vi "valve_test.vi"() -> ()   [LabVIEW 2020]
uses:
  istr.lib/Agilent 33XXX Series/Agilent 33XXX Series.lvlib
panel:
  out "error out":errorcluster
  in  "Amplitude (1)":dbl=1.0
  in  "VISA resource name":refnum<visa-resource-name>
  out "Status":bool
  in  "Interval (s)":dbl
  out "Cycle #":i32
  in  "stop":bool
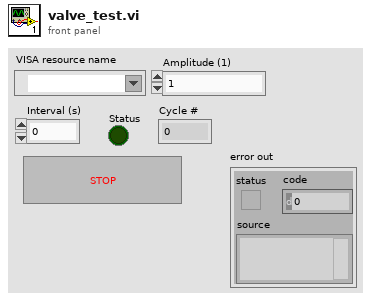
[diagram p1: front panel]
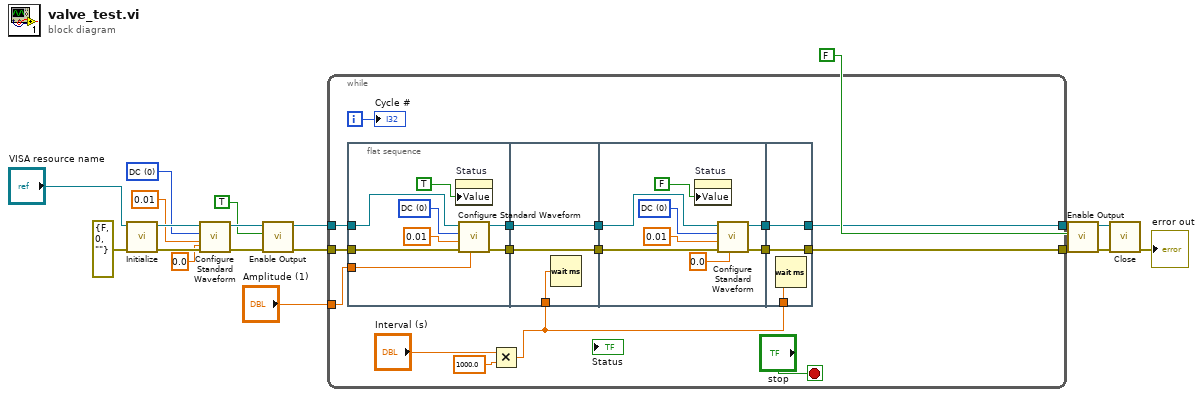
[diagram p0: block diagram]
diagram:
  w13 = u16 0 items=["DC", "Sine", "Square", "Triangle", "Ramp", "Pulse", "Noise", "Sinc", "Negative Ramp", "Exponential Rise", "Exponential Fall", "Cardiac"] ("Waveform Function (1: Sine)")
  n1 = call "Initialize.vi"("error in (no error)"=errorcluster {"status"=FALSE, "code"=0, "source"=""}, "VISA resource name"="VISA resource name") -> ("error out"=w17:errorcluster, "VISA resource name out"=w18:refnum<visa-resource-name>)  [unwired: 8 in]
  n2 = call "Configure Standard Waveform.vi"("DC Offset (0.00 V)"=0.0, "error in (no error)"=w17, "Amplitude (1)"=0.01, "Waveform Function (1: Sine)"=w13, "VISA resource name"=w18) -> ("error out"=w9:errorcluster, "VISA resource name out"=w10:refnum<visa-resource-name>)  [unwired: 5 in]
  n3 = call "Enable Output.vi"("error in (no error)"=w9, "Enable Output  (T: Enable)"=TRUE, "VISA resource name"=w10) -> ("error out"=w6:errorcluster, "VISA resource name out"=w7:refnum<visa-resource-name>)  [unwired: 7 in]
  n4 = while {
    tunnel: "Amplitude (1)" -> [w29]
    tunnel: w7 -> [w28]
    tunnel: w6 -> [w27]
    tunnel: [w24] -> w5
    tunnel: [w23] -> w4
    i -> [w35]
    stop <- "stop" stop-if-true
    n5 = flat-sequence {
      tunnel: [w42] -> w31
      tunnel: w29 -> [w41]
      tunnel: w28 -> [w40]
      tunnel: w27 -> [w39]
      tunnel: [w38] -> w25
      tunnel: w20 -> [w46]
      tunnel: w31 -> [w45]
      tunnel: [w45] -> w30
      tunnel: [w44] -> w26
      tunnel: w25 -> [w44]
      tunnel: w30 -> [w53]
      tunnel: w26 -> [w52]
      tunnel: [w50] -> w22
      tunnel: [w49] -> w21
      tunnel: [w56] -> w23
      tunnel: [w57] -> w24
      tunnel: w22 -> [w57]
      tunnel: w21 -> [w56]
      tunnel: w20 -> [w55]
      frame #0 {
        w36 = u16 0 items=["DC", "Sine", "Square", "Triangle", "Ramp", "Pulse", "Noise", "Sinc", "Negative Ramp", "Exponential Rise", "Exponential Fall", "Cardiac"] ("Waveform Function (1: Sine)")
        n6 = property on="Status" class="Bool (strict)"("Value"=TRUE ("Enable Output  (T: Enable)")) -> ()  [unwired: 2 in, 2 out]
        n7 = call "Configure Standard Waveform.vi"("DC Offset (0.00 V)"=w41, "error in (no error)"=w39, "Amplitude (1)"=0.01, "Waveform Function (1: Sine)"=w36, "VISA resource name"=w40) -> ("error out"=w42:errorcluster, "VISA resource name out"=w38:refnum<visa-resource-name>)  [unwired: 5 in]
      }
      frame #1 {
        n8 = Wait (ms)(milliseconds to wait=w46) -> ()  [unwired: 1 out]
      }
      frame #2 {
        w48 = u16 0 items=["DC", "Sine", "Square", "Triangle", "Ramp", "Pulse", "Noise", "Sinc", "Negative Ramp", "Exponential Rise", "Exponential Fall", "Cardiac"] ("Waveform Function (1: Sine)")
        n9 = property on="Status" class="Bool (strict)"("Value"=FALSE ("Enable Output  (T: Enable)")) -> ()  [unwired: 2 in, 2 out]
        n10 = call "Configure Standard Waveform.vi"("DC Offset (0.00 V)"=0.0, "error in (no error)"=w53, "Amplitude (1)"=0.01, "Waveform Function (1: Sine)"=w48, "VISA resource name"=w52) -> ("error out"=w50:errorcluster, "VISA resource name out"=w49:refnum<visa-resource-name>)  [unwired: 5 in]
      }
      frame #3 {
        n11 = Wait (ms)(milliseconds to wait=w55) -> ()  [unwired: 1 out]
      }
    }
    n12 = Multiply(x="Interval (s)", y=1000.0) -> (x*y=w20:dbl)
    "Cycle #" <- w35
  }
  n13 = call "Enable Output.vi"("error in (no error)"=w5, "Enable Output  (T: Enable)"=FALSE, "VISA resource name"=w4) -> ("error out"=w1:errorcluster, "VISA resource name out"=w2:refnum<visa-resource-name>)  [unwired: 7 in]
  n14 = call "Close.vi"("error in (no error)"=w1, "VISA resource name"=w2) -> ("error out"=→"error out":errorcluster)  [unwired: 9 in]
